vi "Init_Test.vi"(8 "error in (no error)":errorcluster caption="entrée d'erreur (pas d'erreur)", 11 "Delay en entrée":refnum<class "P1833_Scan_QRCode.lvclass">) -> (0 "error out":errorcluster caption="sortie d'erreur", 3 "Delay en sortie":refnum<class "P1833_Scan_QRCode.lvclass">)   [LabVIEW 2020, in "Library Test.lvlib" / "P1833_Scan_QRCode.lvclass"]
uses:
  P1833_Scan_QRCode.lvclass
  C:/Users/ngarcin/OneDrive - Altyor/Standard TB/Class/Test/Test (Default)/Test (Default).lvclass
  Commun VI/TypeDef/Commande Test/Commande Type Test.ctl
  Commun VI/TypeDef/Commande Test/Commande Value Type.ctl
  Test_Without_Instr/Test_Without_Inst.lvclass
  P1833_Scan_QRCode.lvclass/P1833_Scan_QRCode.ctl
  Commun VI/Library Commun.lvlib
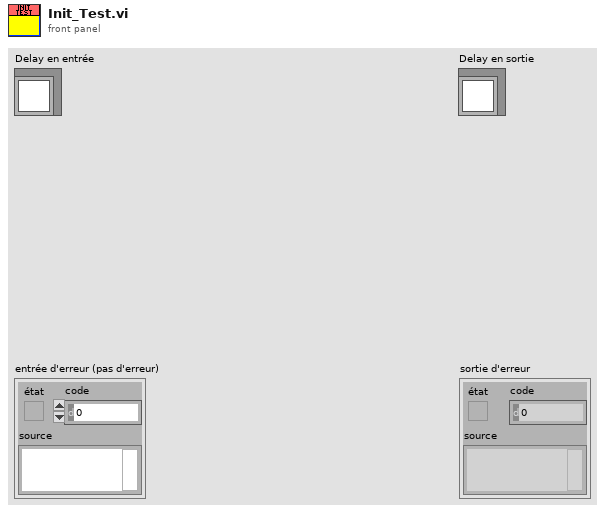
[diagram p1: front panel]
types:
  T1 = typedef "Library Commun.lvlib/Commande Value Type.ctl" = enum16{"None", "String", "Number", "Timestamp", "Boolean", "Array"}
  T2 = typedef "Library Commun.lvlib/Commande Type Test.ctl" = enum16{"Function", "Test", "Calculation"}
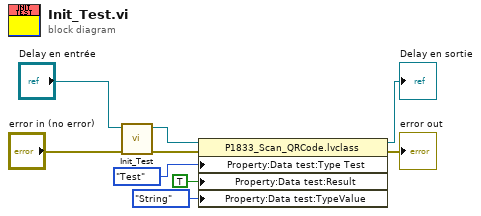
[diagram p0: block diagram]
diagram:
  n1 = call-parent "Init_Test.vi"("error in (no error)"="error in (no error)", "Test_Without_Inst en entrée"="Delay en entrée") -> ("error out"=w6:errorcluster, "Test_Without_Inst en sortie"=w7:refnum<class "P1833_Scan_QRCode.lvclass">)  [unwired: 8 in]
  n2 = property class="P1833_Scan_QRCode.lvclass"(reference=w7, error in=w6, "Property:Data test:Type Test"=Commande_Type_Test."Test" ("Type Test"), "Property:Data test:Result"=TRUE ("Result"), "Property:Data test:TypeValue"=Commande_Value_Type."String" ("TypeValue")) -> (reference out=→"Delay en sortie":refnum<class "P1833_Scan_QRCode.lvclass">, error out=→"error out":errorcluster)
